vi "VIP Publish UI.vi"() -> ()   [LabVIEW 2014, in "VIP Publish Node.lvclass"]
uses:
  VIP Publish Node.lvclass
  <vilib>/NI/Configuration Framework/Node/NodeRef.ctl
  <vilib>/ni/Configuration Framework/Node/NISE_CEF_Node.lvclass
  <vilib>/NI/AMC/Message Queue.ctl
  <vilib>/NI/AMC/Message.ctl
  <vilib>/NI/Tools/Keyed Array/KeyedArray.ctl
  <vilib>/NI/Configuration Framework/Node/UserEventRef.ctl
  <vilib>/NI/Configuration Framework/Controls/EventCluster.ctl
  VIP Publish Node.lvclass/VIP Publish Node.ctl
  Classes/Build Job/Build Job.lvclass/Build Job.ctl
  <vilib>/NI/AMC/Create Single Message.vi
  <vilib>/NI/AMC/Update Message Routing Info.vi
  <vilib>/NI/AMC/Send Message.vi
  Classes/Build Job/Build Job.lvclass
  <vilib>/NI/AMC/AMC.lvlib
  <vilib>/NI/Tools/Keyed Array/Tools_KeyedArray.lvlib
  <vilib>/NI/Configuration Framework/NISE_CEF_TreeControl.lvlib
panel:
  in  "Repo Name":string
  in  "user event":T1
  in  "main queue":T2
  in  "VI Package Path":path=path "C:/Projects/LabVIEW Continuous Integration/LabVIEW Continuous Integration.lvproj"
  in  "Description":string
  in  "node ref":T3
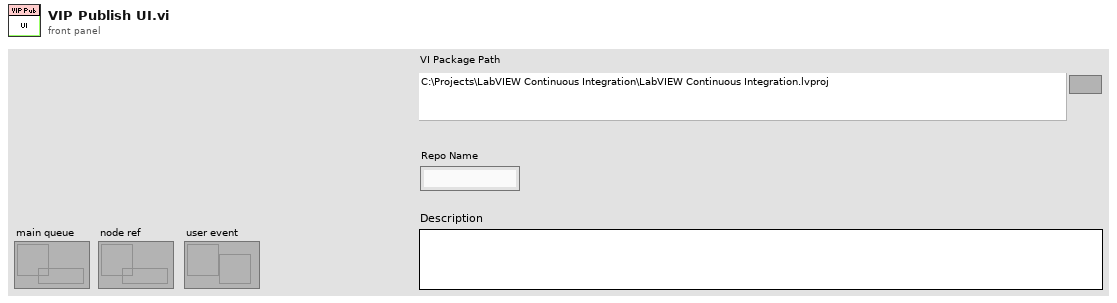
[diagram p1: front panel]
types:
  T1 = typedef "NISE_CEF_Node.lvclass/UserEventRef.ctl" = refnum<user-event>
  T2 = typedef "AMC.lvlib/Message Queue.ctl" = refnum<queue>
  T3 = typedef "NISE_CEF_Node.lvclass/NodeRef.ctl" = refnum<data-value>
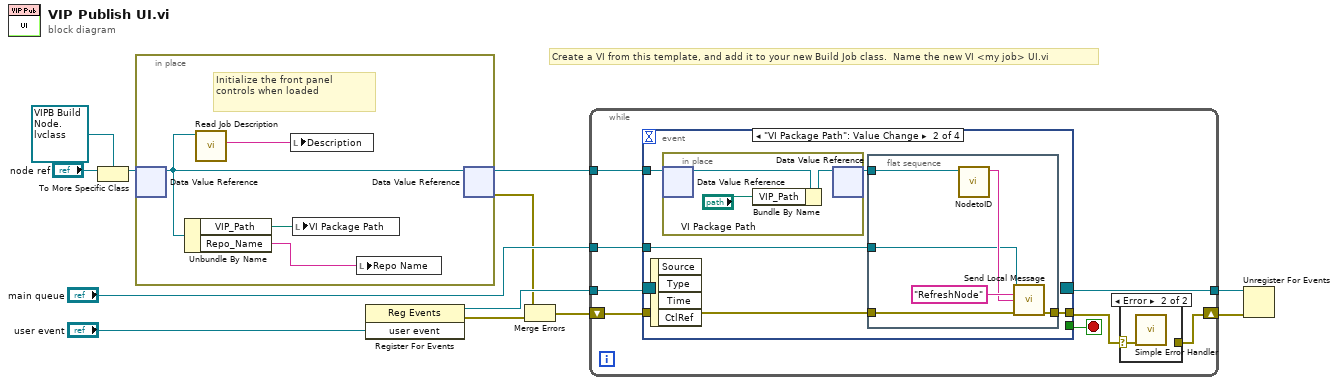
[diagram p0: block diagram]
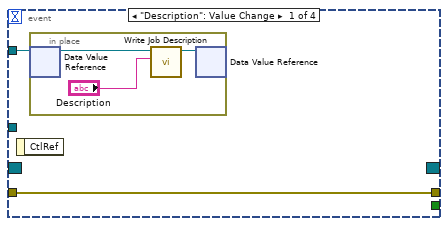
[diagram p3: hidden frame]
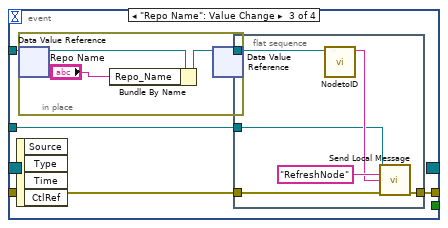
[diagram p4: hidden frame]
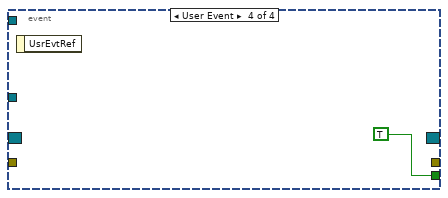
[diagram p5: hidden frame]
diagram:
  # "Create a VI from this template, and add it to your new Build Job class.  Name the new VI <my job> UI.vi"
  n1 = To More Specific Class(target class=refnum<data-value> refnum ("data value reference"), reference="node ref") -> (specific class reference=w6:refnum<data-value>)  [unwired: 1 in, 1 out]
  n2 = in-place {
    # "Initialize the front panel controls when loaded"
    n3 = in-place-dvr #1(w6) -> (w15:refnum<class "VIP Publish Node.lvclass">)  [unwired: 1 out]
    n4 = Unbundle By Name(w15) -> ("VIP_Path"=w14:path, "Repo_Name"=w13:string)
    n5 = call-dynamic "Read Job Description.vi"("Build Job in"=w15) -> ("Job Description"=w16:string)  [unwired: 10 in]
    n6 = local write "Description"(w16) -> ()
    n7 = local write "VI Package Path"(w14) -> ()
    n8 = local write "Repo Name"(w13) -> ()
    n9 = in-place-dvr #1(w15) -> (w2:refnum<data-value>, w4:errorcluster)
  }
  n10 = register-events("user event") -> (reference out=w10:refnum<event-registration>, error out=w5:errorcluster)  [unwired: 2 in]
  n11 = Merge Errors(w4, w5) -> (w3:errorcluster)
  n12 = while {
    tunnel: w2 -> [w24]
    tunnel: "main queue" -> [w23]
    tunnel: w10 -> [w22]
    tunnel: [w21] -> w9
    shift-right: [w17] -> w8
    shift-left: w3 -> [w20]
    stop <- w19 stop-if-true
    n13 = event shown="[1] \"VI Package Path\": Value Change" {
      selector: w22 -> [_ _ _ _]
      dyn-events: [_ _ _ _] -> w21
      timeout: _ -> [_ _ _ _]
      tunnel: w24 -> [w28 w36 w50 _]
      tunnel: w23 -> [_ w32 w46 _]
      tunnel: [_ _ _ TRUE] -> w19
      tunnel: [w27 w33 w47 _] -> w18
      tunnel: w20 -> [w27 w34 w48 _]
      event "Description": Value Change {
        n14 = event-data() -> ()  [unwired: 1 in, 1 out]
        n15 = in-place {
          n16 = in-place-dvr #2(w28) -> (w31:refnum<class "VIP Publish Node.lvclass">)  [unwired: 1 out]
          n17 = call "Write Job Description.vi"("Job Description"="Description", "Build Job in"=w31) -> ("Build Job out"=w30:refnum<class "VIP Publish Node.lvclass">)  [unwired: 9 in]
          n18 = in-place-dvr #2(w30) -> ()  [unwired: 2 out]
        }
      }
      event "VI Package Path": Value Change {
        n19 = event-data() -> ()  [unwired: 1 in, 4 out]
        n20 = in-place {
          n21 = in-place-dvr #3(w36) -> (w45:refnum<class "VIP Publish Node.lvclass">)  [unwired: 1 out]
          n22 = Bundle By Name(cluster=w45, "VIP_Path"="VI Package Path") -> (w44:refnum<class "VIP Publish Node.lvclass">)
          n23 = in-place-dvr #3(w44) -> (w35:refnum<data-value>)  [unwired: 1 out]
        }
        n24 = flat-sequence {
          tunnel: w35 -> [w40]
          tunnel: w34 -> [w39]
          tunnel: [w38] -> w33
          tunnel: w32 -> [w37]
          frame #0 {
            n25 = call <vilib>:"NodetoID.vi"("node ref"=w40) -> ("ID"=w41:string)  [unwired: 9 in, 1 out]
            n26 = call <vilib>:"Send Local Message.vi"("message queue in"=w37, "message name"="RefreshNode" ("Message Name"), "message value"=w41, "error in"=w39) -> ("error out"=w38:errorcluster)  [unwired: 9 in, 2 out]
          }
        }
      }
      event "Repo Name": Value Change {
        n27 = event-data() -> ()  [unwired: 1 in, 4 out]
        n28 = in-place {
          n29 = in-place-dvr #4(w50) -> (w59:refnum<class "VIP Publish Node.lvclass">)  [unwired: 1 out]
          n30 = Bundle By Name(cluster=w59, "Repo_Name"="Repo Name") -> (w58:refnum<class "VIP Publish Node.lvclass">)
          n31 = in-place-dvr #4(w58) -> (w49:refnum<data-value>)  [unwired: 1 out]
        }
        n32 = flat-sequence {
          tunnel: w49 -> [w54]
          tunnel: w48 -> [w53]
          tunnel: [w52] -> w47
          tunnel: w46 -> [w51]
          frame #0 {
            n33 = call <vilib>:"NodetoID.vi"("node ref"=w54) -> ("ID"=w55:string)  [unwired: 9 in, 1 out]
            n34 = call <vilib>:"Send Local Message.vi"("message queue in"=w51, "message name"="RefreshNode" ("Message Name"), "message value"=w55, "error in"=w53) -> ("error out"=w52:errorcluster)  [unwired: 9 in, 2 out]
          }
        }
      }
      event User Event {
        n35 = event-data() -> ()  [unwired: 1 in, 1 out]
      }
    }
    n36 = case shown="Error" w18 {
      selector: w18 -> [w25 w26]
      tunnel: [w25 _] -> w17
      frame No Error {
      }
      frame Error {
        n37 = call <vilib>:"Simple Error Handler.vi"("error in (no error)"=w26) -> ()  [unwired: 4 in, 5 out]
      }
    }
  }
  n38 = Unregister For Events(event registration refnum=w9, error in=w8) -> ()  [unwired: 1 out]
